vi "Update Plot Color.vi"(8 "error in (no error)":errorcluster, 9 "Color":u32(colorbox), 10 "Index":i32, 11 "HistorianCharting in":refnum<class "HistorianCharting.lvclass">) -> (0 "error out":errorcluster, 3 "HistorianCharting out":refnum<class "HistorianCharting.lvclass">)   [LabVIEW 2020, in "VolatusGUIElements.lvlib" / "HistorianCharting.lvclass"]
uses:
  HistorianCharting.lvclass
  HistorianCharting.lvclass/HistorianCharting.ctl
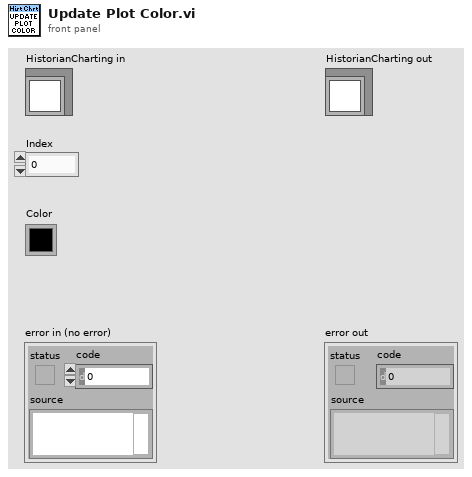
[diagram p1: front panel]
types:
  T1 = typedef "VolatusGUI.lvlib/Historian Charting Manager.lvclass/Plot Config.ctl" = cluster{"Channel":string, "Visible":bool, "Color":u32, "Scale":T2}
  T2 = typedef "VolatusGUI.lvlib/Historian Charting Manager.lvclass/Scale.ctl" = enum16{"Left", "Right"}
  T3 = typedef "VolatusGUI.lvlib/Historian Charting Manager.lvclass/Plot Group Config.ctl" = cluster{"Name":string, "X-Axis Type":T4, "X-Axis Channel":string, "Plots":T1[], "Lock Now":bool, "Time":string, "Swap Axes":bool}
  T4 = typedef "VolatusGUI.lvlib/Historian Charting Manager.lvclass/X-Axis Type.ctl" = enum16{"Time", "Channel"}
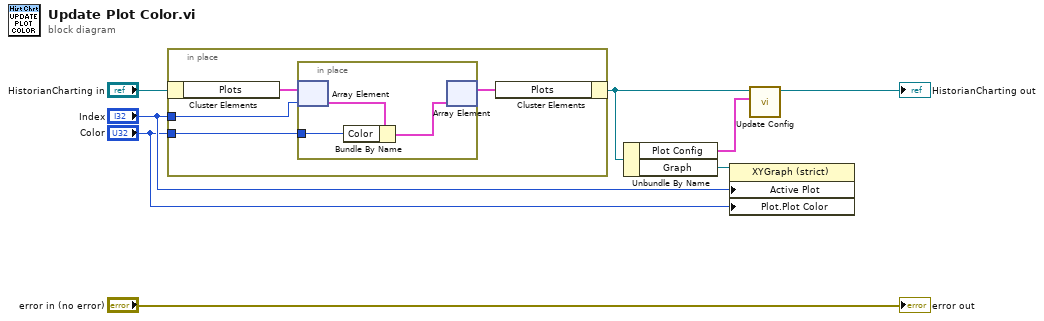
[diagram p0: block diagram]
diagram:
  n1 = in-place {
    in-place-border: "Index" -> [w11]
    in-place-border: "Color" -> [w10]
    n2 = in-place-cluster #1("HistorianCharting in") -> ("Plots"=w12:T1[])
    n3 = in-place {
      in-place-border: w10 -> [w14]
      n4 = in-place-array #2(w12, w11) -> (w15:T1)
      n5 = Bundle By Name(cluster=w15, "Color"=w14) -> (w13:T1)
      n6 = in-place-array #2(w13) -> (w9:T1[])  [unwired: 1 out]
    }
    n7 = in-place-cluster #1("Plots"=w9) -> (w6:refnum<class "HistorianCharting.lvclass">)
  }
  n8 = Unbundle By Name(w6) -> ("Plot Config"=w1:T3, "Graph"=w5:refnum<vi>)
  n9 = property class="XYGraph (strict)"(reference=w5, "Active Plot"="Index", "Plot.Plot Color"="Color") -> ()  [unwired: 1 in, 2 out]
  n10 = call "Update Config.vi"("Config"=w1, "HistorianCharting in"=w6) -> ("HistorianCharting out"=→"HistorianCharting out":refnum<class "HistorianCharting.lvclass">)  [unwired: 8 in, 1 out]
  "error out" <- "error in (no error)"
